vi "Write VISA Port.vi"(8 "error in (no error)":errorcluster, 10 "VISA Port":string, 11 "RS232_Device in":refnum<class "RS232_Device.lvclass">) -> (0 "error out":errorcluster, 3 "RS232_Device out":refnum<class "RS232_Device.lvclass">)   [LabVIEW 2023, in "RS232_Device.lvclass"]
uses:
  RS232_Device.lvclass
  RS232_Device.lvclass/RS232_Device.ctl
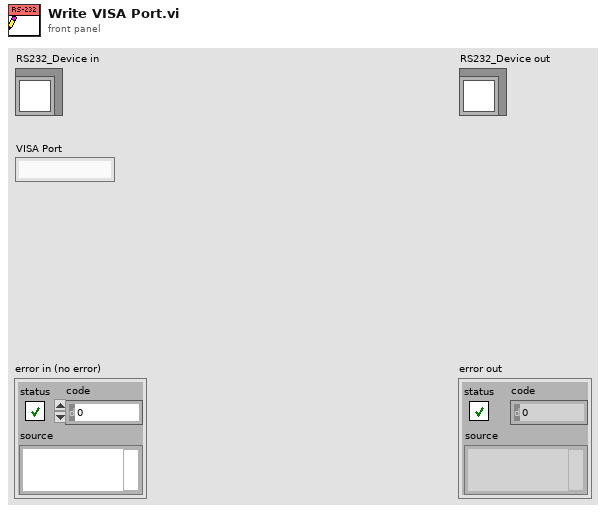
[diagram p1: front panel]
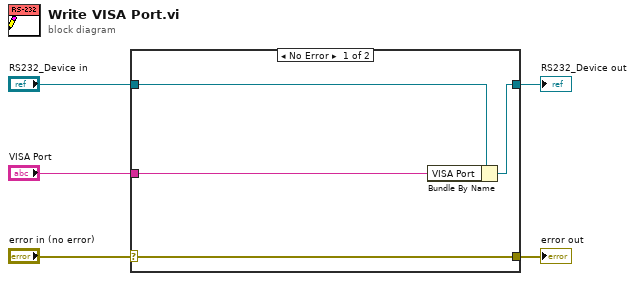
[diagram p0: block diagram]
diagram:
  n1 = case shown="No Error" "error in (no error)" {
    selector: "error in (no error)" -> [w9 w10]
    tunnel: [w9 w10] -> w4
    tunnel: [w7 w11] -> w2
    tunnel: "RS232_Device in" -> [w8 w11]
    tunnel: "VISA Port" -> [w6 _]
    frame No Error {
      n2 = Bundle By Name(cluster=w8, "VISA Port"=w6) -> (w7:refnum<class "RS232_Device.lvclass">)
    }
    frame Error {
    }
  }
  "error out" <- w4
  "RS232_Device out" <- w2
